vi "Trigger.vi"(0 "Lines":tag="Dev1/port1/line0:1, Dev1/port1/line3:7", 1 "Line2":tag="Dev1/port1/line2" caption="Line2: ISS Data Acquisition Done Signal", 2 "Delaytime(ms)":u32=200, 3 "Turn All Lasers OFF":bool[](array[boolean])=[FALSE, FALSE, TRUE, FALSE, FALSE, FALSE, FALSE] caption="Output Data 1", 4 "Milliseconds to wait\nbefore checking MARK":u32, 5 "Turn ISS Lasers ON":bool[](array[boolean])=[FALSE, FALSE, FALSE, FALSE, FALSE, FALSE, FALSE] caption="Output Data 2", 6 "Mark":bool, 7 "Send ISS a Trigger":bool[](array[boolean])=[TRUE, FALSE, FALSE, FALSE, FALSE, FALSE, FALSE] caption="Output Data 3", 9 "Send a Mark Signal\nif MARK is selected":bool[](array[boolean])=[FALSE, FALSE, FALSE, TRUE, FALSE, FALSE, FALSE] caption="Output Data") -> (8 "Input Data":bool=TRUE caption="Feedback")   [LabVIEW 2014]
uses:
  <vilib>/Utility/error.llb/DialogType.ctl
  <vilib>/DAQmx/create/channels.llb/DAQmx Create Channel (DO-Digital Output).vi
  <vilib>/DAQmx/write.llb/DAQmx Write (Digital 1D Bool 1Chan 1Samp).vi
  <vilib>/DAQmx/create/channels.llb/DAQmx Create Channel (DI-Digital Input).vi
  <vilib>/DAQmx/read.llb/DAQmx Read (Digital Bool 1Line 1Point).vi
panel:
  in  "Post ISS Delay (ms)":i32=1000
  out "ISS Laser":bool
  # "Channel Parameters"
  # "Line    Signal\n\n0           ISS Trigger (0: OFF, 1: ON)\n1           Flow Laser 1 ON/OFF (0:OFF, 1:ON)\n2           ISS Data Acquisition (0: DONE, 1: NO)\n3           ISS Laser ON/OFF (0: ON, 1: OFF)\n4           Trigger for Marks  (0: OFF, 1: ON)\n5           Flow Laser 2 ON/OFF (0:OFF, 1:ON)\n6           Reserved\n7           Reserved"
  # "Step1"
  # "Line"
  # "0"
  # "1"
  # "3"
  # "4"
  # "5"
  # "6"
  # "7"
  # "*The number of lines in the list must\nmatch the number of elements in\nthe array."
  # "Step2"
  # "Line"
  # "0"
  # "1"
  # "3"
  # "4"
  # "5"
  # "6"
  # "7"
  # "Step3"
  # "Line"
  # "0"
  # "1"
  # "3"
  # "4"
  # "5"
  # "6"
  # "7"
  # "Step4"
  # "Line"
  # "0"
  # "1"
  # "3"
  # "4"
  # "5"
  # "6"
  # "7"
  # "Step5"
  # "Get ISS Data Acuisition Signal"
  # "Line"
  # "2"
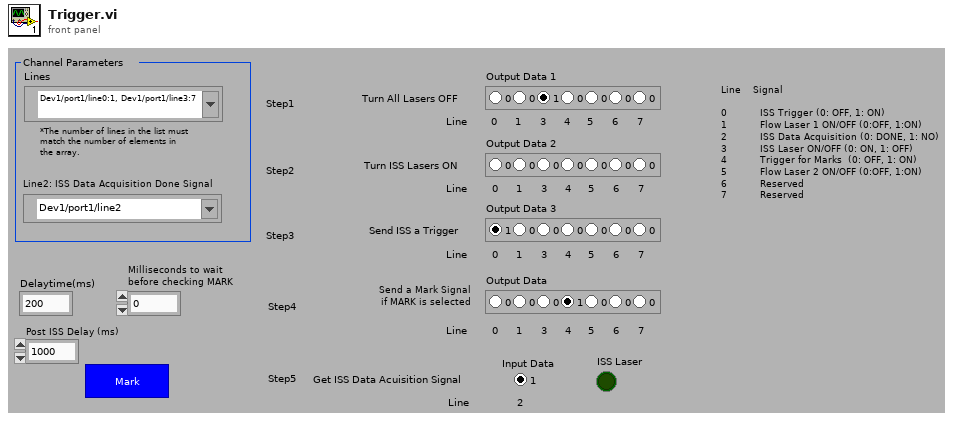
[diagram p1: front panel]
types:
  T1 = typedef "DialogType.ctl" = u16
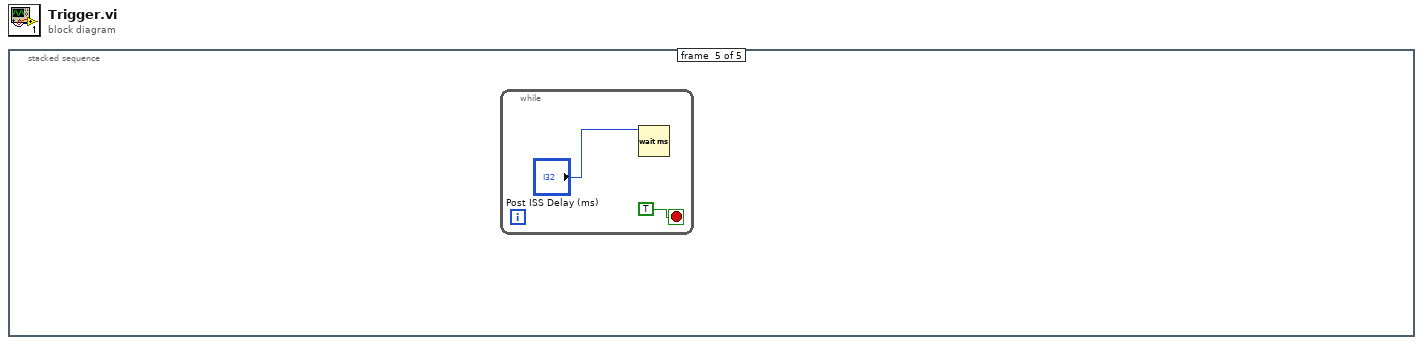
[diagram p0: block diagram]
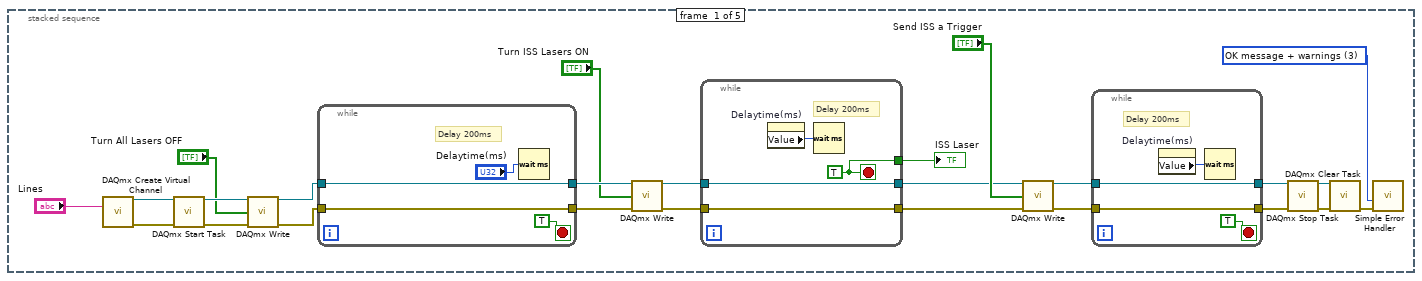
[diagram p2: hidden frame]
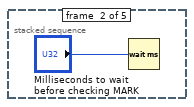
[diagram p3: hidden frame]
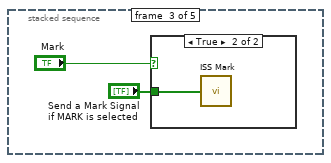
[diagram p4: hidden frame]
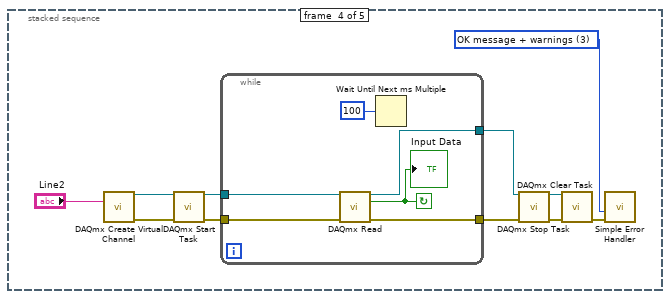
[diagram p6: hidden frame]
diagram:
  n1 = stacked-sequence {
    frame #0 {
      w20 = T1 3 items=["no dialog", "OK message", "continue or stop message", "OK message + warnings", "continue/stop + warnings"] ("type of dialog (OK msg:1)")
      n2 = call-poly <vilib>:"DAQmx Create Virtual Channel.vi"("lines"="Lines") -> ("task out"=w25:refnum<k21>, "error out"=w24:errorcluster)  [unwired: 13 in]
      n3 = call <vilib>:"DAQmx Start Task.vi"("task/channels in"=w25, "error in"=w24) -> ("task out"=w23:refnum<k21>, "error out"=w22:errorcluster)  [unwired: 12 in]
      n4 = call-poly <vilib>:"DAQmx Write.vi"("task/channels in"=w23, "data"="Turn All Lasers OFF", "error in"=w22) -> ("task out"=w18:refnum<k21>, "error out"=w17:errorcluster)  [unwired: 10 in, 1 out]
      n5 = while {
        tunnel: w18 -> [w36]
        tunnel: w17 -> [w35]
        tunnel: [w36] -> w16
        tunnel: [w35] -> w15
        stop <- TRUE stop-if-true
        # "Delay 200ms"
        n6 = Wait (ms)(milliseconds to wait="Delaytime(ms)") -> ()  [unwired: 1 out]
      }
      n7 = call-poly <vilib>:"DAQmx Write.vi"("task/channels in"=w16, "data"="Turn ISS Lasers ON", "error in"=w15) -> ("task out"=w13:refnum<k21>, "error out"=w12:errorcluster)  [unwired: 10 in, 1 out]
      n8 = while {
        tunnel: w13 -> [w33]
        tunnel: w12 -> [w32]
        tunnel: [w33] -> w6
        tunnel: [w32] -> w5
        tunnel: [w30] -> w1
        stop <- w30 stop-if-true
        w30 = TRUE
        # "Delay 200ms"
        n9 = property on="Delaytime(ms)" class="DigNum (strict)"() -> ("Value"=w31:u32)  [unwired: 2 in, 2 out]
        n10 = Wait (ms)(milliseconds to wait=w31) -> ()  [unwired: 1 out]
      }
      "ISS Laser" <- w1
      n11 = call-poly <vilib>:"DAQmx Write.vi"("task/channels in"=w6, "data"="Send ISS a Trigger", "error in"=w5) -> ("task out"=w10:refnum<k21>, "error out"=w9:errorcluster)  [unwired: 10 in, 1 out]
      n12 = while {
        tunnel: w10 -> [w29]
        tunnel: w9 -> [w28]
        tunnel: [w29] -> w8
        tunnel: [w28] -> w7
        stop <- TRUE stop-if-true
        # "Delay 200ms"
        n13 = property on="Delaytime(ms)" class="DigNum (strict)"() -> ("Value"=w27:u32)  [unwired: 2 in, 2 out]
        n14 = Wait (ms)(milliseconds to wait=w27) -> ()  [unwired: 1 out]
      }
      n15 = call <vilib>:"DAQmx Stop Task.vi"("task/channels in"=w8, "error in"=w7) -> ("task out"=w4:refnum<k21>, "error out"=w3:errorcluster)  [unwired: 12 in]
      n16 = call <vilib>:"DAQmx Clear Task.vi"("task in"=w4, "error in"=w3) -> ("error out"=w21:errorcluster)  [unwired: 13 in]
      n17 = call <vilib>:"Simple Error Handler.vi"("type of dialog (OK msg:1)"=w20, "error in (no error)"=w21) -> ()  [unwired: 3 in, 5 out]
    }
    frame #1 {
      n18 = Wait (ms)(milliseconds to wait="Milliseconds to wait\nbefore checking MARK") -> ()  [unwired: 1 out]
    }
    frame #2 {
      n19 = case shown="True" "Mark" {
        tunnel: "Send a Mark Signal\nif MARK is selected" -> [_ w41]
        frame False {
        }
        frame True {
          n20 = call "ISS Mark.vi"("Send a Mark Signal"=w41) -> ()  [unwired: 3 in]
        }
      }
    }
    frame #3 {
      w46 = T1 3 items=["no dialog", "OK message", "continue or stop message", "OK message + warnings", "continue/stop + warnings"] ("type of dialog (OK msg:1)")
      n21 = call-poly <vilib>:"DAQmx Create Virtual Channel.vi"("lines"="Line2") -> ("task out"=w52:refnum<k21>, "error out"=w51:errorcluster)  [unwired: 13 in]
      n22 = call <vilib>:"DAQmx Start Task.vi"("task/channels in"=w52, "error in"=w51) -> ("task out"=w49:refnum<k21>, "error out"=w48:errorcluster)  [unwired: 12 in]
      n23 = while {
        tunnel: w49 -> [w58]
        tunnel: w48 -> [w57]
        tunnel: [w56] -> w43
        tunnel: [w55] -> w42
        stop <- w53 continue-if-true
        n24 = call-poly <vilib>:"DAQmx Read.vi"("task/channels in"=w58, "error in"=w57) -> ("task out"=w56:refnum<k21>, "data"=w53:bool, "error out"=w55:errorcluster)  [unwired: 11 in]
        "Input Data" <- w53
        n25 = Wait Until Next ms Multiple(millisecond multiple=u32 100 ("milliseconds to wait")) -> ()  [unwired: 1 out]
      }
      n26 = call <vilib>:"DAQmx Stop Task.vi"("task/channels in"=w43, "error in"=w42) -> ("task out"=w45:refnum<k21>, "error out"=w44:errorcluster)  [unwired: 12 in]
      n27 = call <vilib>:"DAQmx Clear Task.vi"("task in"=w45, "error in"=w44) -> ("error out"=w47:errorcluster)  [unwired: 13 in]
      n28 = call <vilib>:"Simple Error Handler.vi"("type of dialog (OK msg:1)"=w46, "error in (no error)"=w47) -> ()  [unwired: 3 in, 5 out]
    }
    frame #4 {
      n29 = while {
        stop <- TRUE stop-if-true
        n30 = Wait (ms)(milliseconds to wait="Post ISS Delay (ms)") -> ()  [unwired: 1 out]
      }
    }
  }
